vi "Self-Test Helper.vi"(4 "OK Button":string="OK", 5 "Dialog Message":string="You must disconnect all external I/O signals from the device before you can perform a full self-test.  \n\nAfter you disconnect cables from the device, click OK. If you do not want to perform a full self-test at this time, click Cancel.", 6 "Self-Test Mode (basic)":i32(ring) items=["basic", "intermediate", "full"], 7 "Dialog Title":string="NI System Configuration Self-Test:", 8 "error in (no error)":errorcluster, 10 "Prompt if Full Mode (T)":bool=TRUE, 11 "Resource in":refnum<k20>) -> (0 "error out":errorcluster, 3 "Resource out":u64)   [LabVIEW 2017, in "nisyscfg.lvlib"]
uses:
  <vilib>/nisyscfg/nisyscfg.lvlib
  <resource>/objmgr/nisysapi.rc
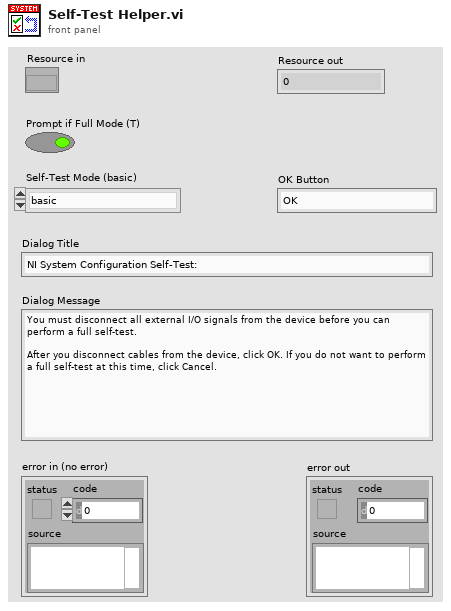
[diagram p1: front panel]
types:
  T1 = enum16{"Left Button", "Center Button", "Right Button", "Window Close"}
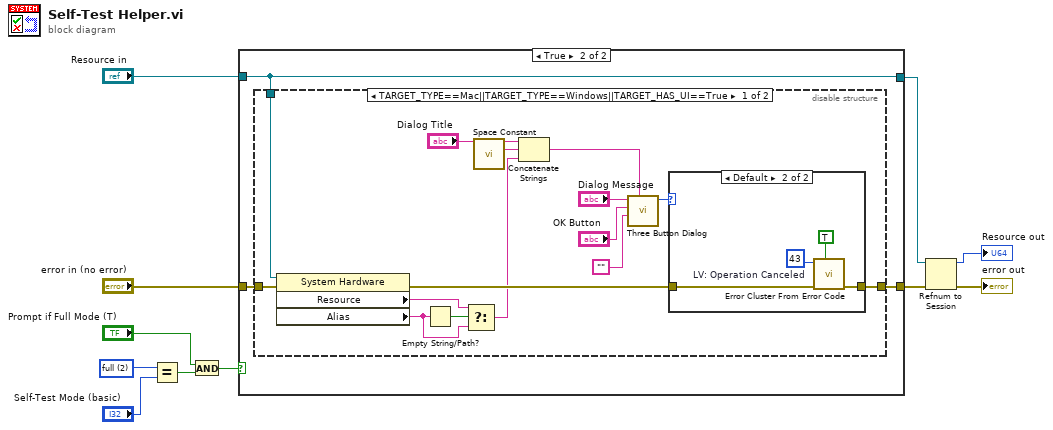
[diagram p0: block diagram]
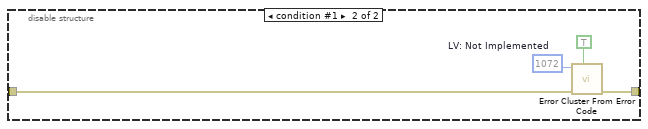
[diagram p4: hidden frame]
diagram:
  w1 = 2 items=["basic", "intermediate", "full"] ("Self-Test Mode (basic) 2")
  n1 = Equal?(x=w1, y="Self-Test Mode (basic)") -> (x = y?=w11:bool)
  n2 = And(x="Prompt if Full Mode (T)", y=w11) -> (x .and. y?=w8:bool)
  n3 = case shown="True" w8 {
    tunnel: "error in (no error)" -> [w13 w15]
    tunnel: [w13 w16] -> w5
    tunnel: "Resource in" -> [w12 w14]
    tunnel: [w12 w14] -> w3
    frame False {
    }
    frame True {
      n4 = disable-structure shown="TARGET_TYPE==Mac||TARGET_TYPE==Windows||TARGET_HAS_UI==True" {
        disable-tunnel: [w26 w38] -> w16
        disable-tunnel: w15 -> [w25 w37]
        disable-tunnel: w14 -> [w23 _]
        frame condition #0 (active) {
          n5 = property class="System Hardware"(reference=w23, error in=w25) -> (error out=w24:errorcluster, "Resource"=w21:string, "Alias"=w20:string)  [unwired: 1 out]
          n6 = Empty String/Path?(string/path=w20) -> (empty?=w22:bool)
          n7 = Select(t=w21, s=w22, f=w20) -> (s? t:f=w17:string)
          n8 = call <vilib>:"Space Constant.vi"() -> ("String"=w18:string)
          n9 = Concatenate Strings("Dialog Title", w18, w17) -> (w19:string)
          n10 = call <vilib>:"Three Button Dialog.vi"("Window Title (\"\")"=w19, "Center Button Text (\"No\")"="", "Left Button Text (\"Yes\")"="OK Button", "message"="Dialog Message") -> ("Which Button?"=w27:T1)  [unwired: 7 in]
          n11 = case shown="Default" w27 {
            tunnel: w24 -> [w32 w35]
            tunnel: [w32 w36] -> w26
            frame "Left Button" {
            }
            frame Default {
              w34 = 43  # LV: Operation Canceled
              n12 = call <vilib>:"Error Cluster From Error Code.vi"("show call chain? (False)"=TRUE, "error in (no error)"=w35, "error code (0)"=w34) -> ("error out"=w36:errorcluster)  [unwired: 6 out]
            }
          }
        }
        frame condition #1 {
          w40 = 1072  # LV: Not Implemented
          n13 = call <vilib>:"Error Cluster From Error Code.vi"("show call chain? (False)"=TRUE, "error in (no error)"=w37, "error code (0)"=w40) -> ("error out"=w38:errorcluster)  [unwired: 6 out]
        }
      }
    }
  }
  n14 = Refnum to Session(4:w5, 7:w3) -> (0:→"error out":errorcluster, 3:→"Resource out":u64)
